vi "niFpgaMeanVarStdInsideSCTL.vi"(0 "input data":fxp<+/-,32,1>, 1 "reset":bool, 9 "input valid":bool, 12 "ready for output":bool=TRUE) -> (4 "mean":fxp<+/-,32,1> format="%.32g", 6 "standard deviation":fxp<+,32,1> format="%.32g", 8 "variance":fxp<+,63,1> format="%.63g", 10 "output valid":bool, 14 "ready for input":bool)   [LabVIEW 2017]
uses:
  <vilib>/rvi/FXPMathLib/basic elements/FxpIntAccumulator/subVIs/nifxpmath_IntAccumulator_SimConfig.ctl
  <vilib>/rvi/FXPMathLib/basic elements/FxpIntAccumulator/simVIs/DllFxpIntAccumulator_sub.vi
  <vilib>/rvi/FXPMathLib/basic elements/FxpIntAccumulator/XNode/nifxpmath_IntAccumulator.xnode
  <vilib>/fxp/LVFixedPointOverflowPolicyTypeDef.ctl
  <vilib>/rvi/FXPMathLib/FxpMul/XNode/nifxpmath_Multiplier.xnode
  <vilib>/rvi/FXPMathLib/FxpSqrt/XNode/nifxpmath_Sqrt.xnode
  <vilib>/rvi/FXPMathLib/FxpSqrt/simVIs/DllSqrtTemp_sub.vi
  <vilib>/rvi/FXPMathLib/FxpSqrt/subVIs/nifxpmath_Sqrt_SimConfig.ctl
  <vilib>/rvi/FXPMathLib/sim/FxpSim.dll
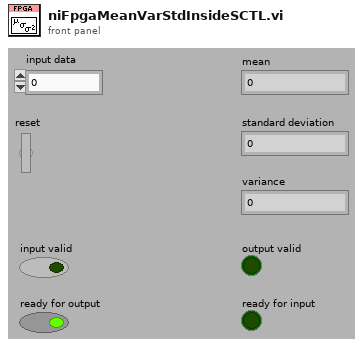
[diagram p1: front panel]
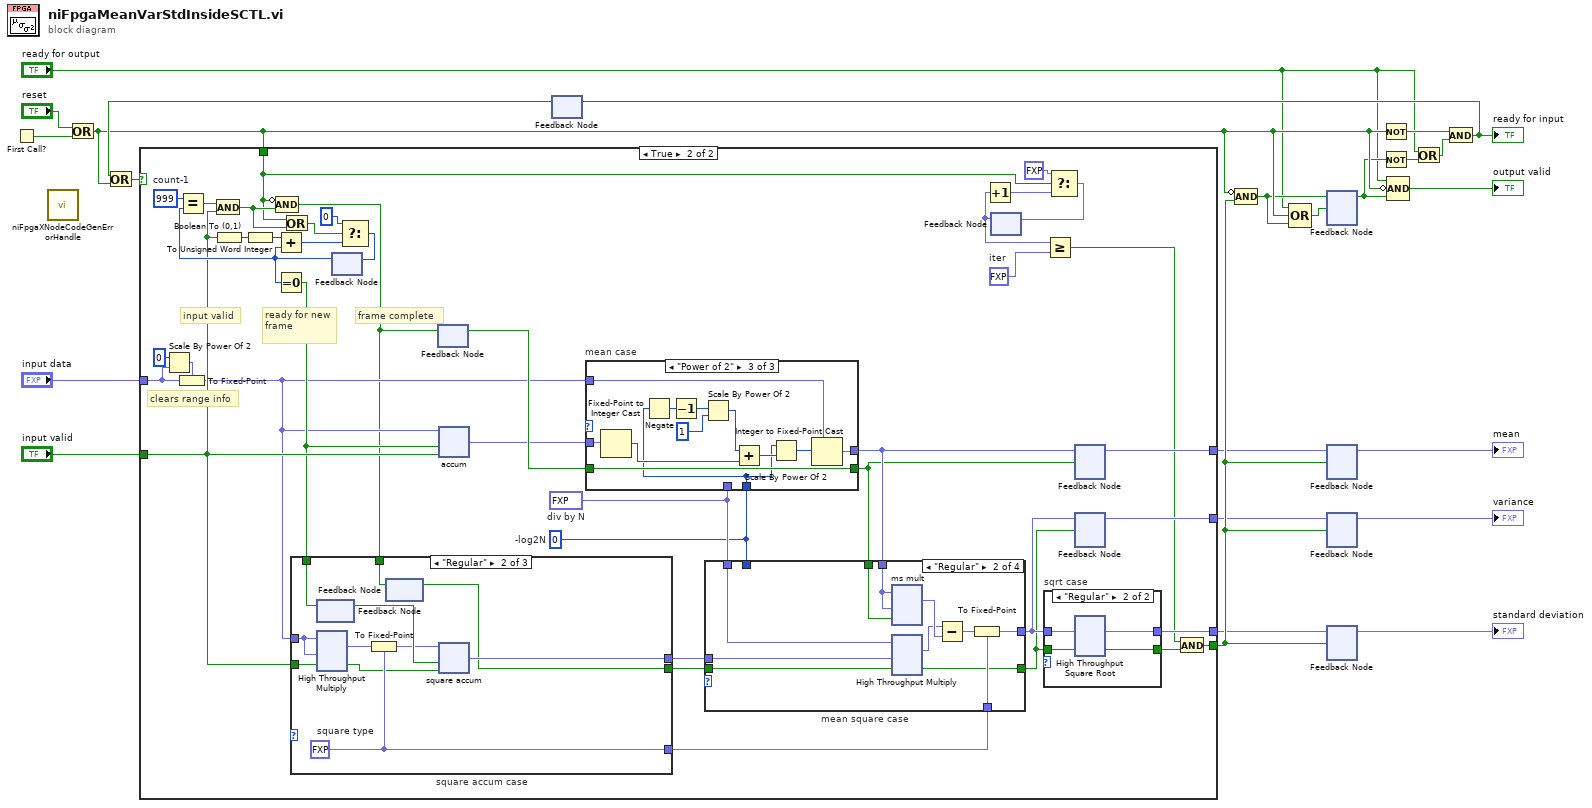
[diagram p0: block diagram]
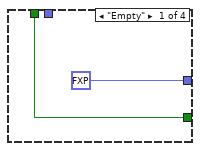
[diagram p3: hidden frame]
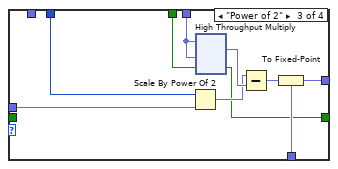
[diagram p4: hidden frame]
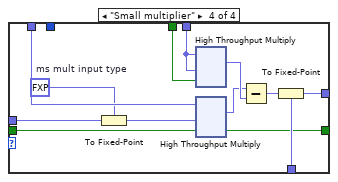
[diagram p5: hidden frame]
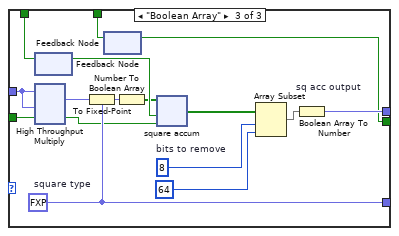
[diagram p7: hidden frame]
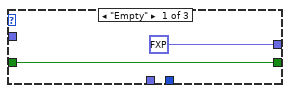
[diagram p8: hidden frame]
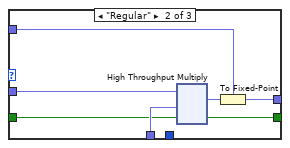
[diagram p9: hidden frame]
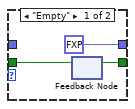
[diagram p10: hidden frame]
diagram:
  n1 = First Call?() -> (First Call?: T/F=w21:bool)
  n2 = call <vilib>:"niFpgaXNodeCodeGenErrorHandle.vi"() -> ()  [unwired: 1 in]
  n3 = Or(x="reset", y=w21) -> (x .or. y?=w7:bool)
  n4 = feedback #1() -> (w9:bool)  [unwired: 1 in]
  n5 = Or(x=w9, y=w7) -> (x .or. y?=w10:bool)
  n6 = case shown="True" w10 {
    tunnel: "input valid" -> [_ w56]
    tunnel: w7 -> [_ w49]
    tunnel: [_ w28] -> w15
    tunnel: [_ w43] -> w14
    tunnel: [_ w42] -> w13
    tunnel: [_ w36] -> w12
    tunnel: "input data" -> [_ w24]
    frame False {
    }
    frame True {
      w35 = i8 0  # -log2N
      w51 = fxp<+,6,6> 39.0  # iter
      w41 = fxp<+,18,-9> 0.0010000020265579224  # div by N
      w47 = u16 999  # count-1
      # "clears range info"
      # "frame complete"
      # "ready for new frame"
      # "input valid"
      n7 = Scale By Power Of 2(n=0, x=w24) -> (x*2^n=w25:fxp<+/-,32,1>)
      n8 = To Fixed-Point(fixed-point type=w25, number=w24) -> (fixed-point=w34:fxp<+/-,32,1>)
      n9 = Boolean To (0,1)(Boolean=w56) -> (0, 1=w63:i16)
      n10 = To Unsigned Word Integer(number=w63) -> (unsigned 16bit integer=w46:u16)
      n11 = feedback #2() -> (w59:u16)  [unwired: 1 in]
      n12 = Equal?(x=w47, y=w59) -> (x = y?=w61:bool)
      n13 = And(x=w61, y=w56) -> (x .and. y?=w57:bool)
      n14 = Compound Arithmetic op=AND(invert w49, w57) -> (w30:bool)
      n15 = Add(x=w46, y=w59) -> (x+y=w62:u16)
      n16 = Equal To 0?(x=w59) -> (x = 0?=w55:bool)
      n17 = Or(x=w49, y=w57) -> (x .or. y?=w58:bool)
      n18 = case "square accum case" shown="\"Regular\"" {
        selector: _ -> [_ _ _]
        tunnel: w56 -> [_ w137 w180]
        tunnel: w55 -> [_ w136 w179]
        tunnel: w34 -> [_ w135 w178]
        tunnel: [_ w134 w177] -> w45
        tunnel: [_ w127 w165] -> w40
        tunnel: [_ w129 w167] -> w39
        tunnel: w30 -> [_ w128 w166]
        frame "Empty" {
        }
        frame "Regular" {
          w134 = fxp<+,31,1> 0.0  # square type
          n19 = feedback-in #3(w136) -> ()
          n20 = feedback #3() -> (w132:bool)  [unwired: 1 in]
          n21 = xnode "High Throughput Multiply"("x"=w135, "y"=w135, "input valid"=w137) -> ("x*y"=w131:fxp<+/-,64,2>, "output valid"=w133:bool)  [unwired: 1 in, 1 out]
          n22 = To Fixed-Point(fixed-point type=w134, number=w131) -> (fixed-point=w130:fxp<+,31,1>)
          n23 = feedback-in #4(w128) -> ()
          n24 = feedback #4() -> (w127:bool)  [unwired: 1 in]
          n25 = xnode "square accum"("x"=w130, "load (F)"=w132, "enable (T)"=w133) -> ("s"=w129:fxp<+,41,11>)  [unwired: 2 in, 1 out]
        }
        frame "Boolean Array" {
          w171 = 8  # bits to remove
          w177 = fxp<+,63,1> 0.0  # square type
          n26 = feedback-in #5(w179) -> ()
          n27 = feedback #5() -> (w175:bool)  [unwired: 1 in]
          n28 = xnode "High Throughput Multiply"("x"=w178, "y"=w178, "input valid"=w180) -> ("x*y"=w174:fxp<+/-,64,2>, "output valid"=w176:bool)  [unwired: 1 in, 1 out]
          n29 = To Fixed-Point(fixed-point type=w177, number=w174) -> (fixed-point=w173:fxp<+,63,1>)
          n30 = feedback-in #6(w166) -> ()
          n31 = feedback #6() -> (w165:bool)  [unwired: 1 in]
          n32 = Number To Boolean Array(number=w173) -> (Boolean array=w172:bool[])
          n33 = xnode "square accum"("x"=w172, "load (F)"=w175, "enable (T)"=w176) -> ("s"=w168:bool[])  [unwired: 2 in, 1 out]
          n34 = Array Subset(array=w168, index=w171, length=64) -> (w169:bool[])
          n35 = Boolean Array To Number "sq acc output"(Boolean array=w169) -> (number=w167:fxp<+,64,10>)
        }
      }
      n36 = Select(t=u16 0, s=w58, f=w62) -> (s? t:f=w48:u16)
      n37 = feedback-in #2(w48) -> ()
      n38 = feedback-in #7(w30) -> ()
      n39 = feedback #7() -> (w38:bool)  [unwired: 1 in]
      n40 = xnode "accum"("x"=w34, "load (F)"=w55, "enable (T)"=w56) -> ("s"=w37:fxp<+/-,42,11>)  [unwired: 2 in, 1 out]
      n41 = case "mean case" shown="\"Power of 2\"" {
        selector: _ -> [_ _ _]
        tunnel: w34 -> [_ w211 w213]
        tunnel: w41 -> [_ w210 _]
        tunnel: w38 -> [w204 w209 w223]
        tunnel: w37 -> [_ w208 w215]
        tunnel: [w204 w207 w223] -> w31
        tunnel: [fxp<+/-,16,1> 0.0 ("input data") w206 w214] -> w32
        tunnel: w35 -> [_ _ w212]
        frame "Empty" {
        }
        frame "Regular" {
          n42 = xnode "High Throughput Multiply"("x"=w208, "y"=w210, "input valid"=w209) -> ("x*y"=w205:fxp<+/-,60,2>, "output valid"=w207:bool)  [unwired: 1 in, 1 out]
          n43 = To Fixed-Point(fixed-point type=w211, number=w205) -> (fixed-point=w206:fxp<+/-,32,1>)
        }
        frame "Power of 2" {
          n44 = Fixed-Point to Integer Cast(1:w215) -> (0:w218:i64)
          n45 = Negate(x=w212) -> (-x=w222:i8)
          n46 = Decrement(x=w222) -> (x-1=w221:i8)
          n47 = Scale By Power Of 2(n=w221, x=i64 1 ("x-1")) -> (x*2^n=w219:i64)
          n48 = Add(x=w219, y=w218) -> (x+y=w216:i64)
          n49 = Scale By Power Of 2(n=w212, x=w216) -> (x*2^n=w217:i64)
          n50 = Integer to Fixed-Point Cast(fixed-point type=w213, integer=w217) -> (fixed-point=w214:fxp<+/-,32,1>)
        }
      }
      n51 = case "mean square case" shown="\"Regular\"" {
        selector: _ -> [_ _ _ _]
        tunnel: w45 -> [_ w103 w113 w126]
        tunnel: [w91 w102 w104 w125] -> w33
        tunnel: [fxp<+,31,1> 0.0 ("square type") w101 w112 w124] -> w44
        tunnel: w41 -> [_ w100 _ w123]
        tunnel: w40 -> [_ w99 _ w122]
        tunnel: w39 -> [_ w98 w111 w121]
        tunnel: w35 -> [_ _ w110 _]
        tunnel: w32 -> [_ w93 w108 w118]
        tunnel: w31 -> [w91 w94 w109 w117]
        frame "Empty" {
        }
        frame "Regular" {
          n52 = xnode ("ms mult")("x"=w93, "y"=w93, "input valid"=w94) -> ("x*y"=w97:fxp<+/-,64,2>)  [unwired: 1 in, 2 out]
          n53 = xnode ("High Throughput Multiply")("x"=w100, "y"=w98, "input valid"=w99) -> ("x*y"=w96:fxp<+,64,2>, "output valid"=w102:bool)  [unwired: 1 in, 1 out]
          n54 = Subtract(x=w96, y=w97) -> (x-y=w95:fxp<+/-,64,4>)
          n55 = To Fixed-Point(fixed-point type=w103, number=w95) -> (fixed-point=w101:fxp<+,63,1>)
        }
        frame "Power of 2" {
          n56 = Scale By Power Of 2(n=w110, x=w111) -> (x*2^n=w106:fxp<+,64,11>)
          n57 = xnode "High Throughput Multiply"("x"=w108, "y"=w108, "input valid"=w109) -> ("x*y"=w107:fxp<+/-,64,2>, "output valid"=w104:bool)  [unwired: 1 in, 1 out]
          n58 = Subtract(x=w106, y=w107) -> (x-y=w105:fxp<+/-,64,13>)
          n59 = To Fixed-Point(fixed-point type=w113, number=w105) -> (fixed-point=w112:fxp<+,63,1>)
        }
        frame "Small multiplier" {
          w119 = fxp<+,34,10> 0.0  # ms mult input type
          n60 = To Fixed-Point(fixed-point type=w119, number=w121) -> (fixed-point=w120:fxp<+,34,10>)
          n61 = xnode ("High Throughput Multiply")("x"=w118, "y"=w118, "input valid"=w117) -> ("x*y"=w116:fxp<+/-,64,2>)  [unwired: 1 in, 2 out]
          n62 = xnode ("High Throughput Multiply")("x"=w123, "y"=w120, "input valid"=w122) -> ("x*y"=w115:fxp<+,52,1>, "output valid"=w125:bool)  [unwired: 1 in, 1 out]
          n63 = Subtract(x=w115, y=w116) -> (x-y=w114:fxp<+/-,64,3>)
          n64 = To Fixed-Point(fixed-point type=w126, number=w114) -> (fixed-point=w124:fxp<+,63,1>)
        }
      }
      n65 = feedback #8() -> (w50:fxp<+,6,6>)  [unwired: 1 in]
      n66 = Increment(x=w50) -> (x+1=w53:fxp<+,6,6>)
      n67 = case "sqrt case" shown="\"Regular\"" {
        selector: _ -> [_ _]
        tunnel: [w224 w230] -> w29
        tunnel: w33 -> [w225 w229]
        tunnel: w44 -> [_ w228]
        tunnel: [fxp<+,16,1> 0.0 ("sqrt(x)") w227] -> w42
        frame "Empty" {
          n68 = feedback-in #9(w225) -> ()
          n69 = feedback #9() -> (w224:bool)  [unwired: 1 in]
        }
        frame "Regular" {
          n70 = xnode ("High Throughput Square Root")("x"=w228, "input valid"=w229) -> ("sqrt(x)"=w227:fxp<+,32,1>, "output valid"=w230:bool)  [unwired: 1 in, 1 out]
        }
      }
      n71 = Greater Or Equal?(x=w50, y=w51) -> (x >= y?=w27:bool)
      n72 = Select(t=fxp<+,1,1> 0.0, s=w49, f=w53) -> (s? t:f=w52:fxp<+,6,6>)
      n73 = feedback-in #8(w52) -> ()
      n74 = feedback-in #10(w32, w31) -> ()
      n75 = feedback #10() -> (w36:fxp<+/-,32,1>)  [unwired: 1 in]
      n76 = feedback-in #11(w44, w33) -> ()
      n77 = feedback #11() -> (w43:fxp<+,63,1>)  [unwired: 1 in]
      n78 = And(x=w27, y=w29) -> (x .and. y?=w28:bool)
    }
  }
  n79 = Compound Arithmetic op=AND(invert w7, w15) -> (w6:bool)
  n80 = Compound Arithmetic op=OR("ready for output", w7, w6) -> (w5:bool)
  n81 = feedback-in #12(w6, w5) -> ()
  n82 = feedback #12() -> (w4:bool)  [unwired: 1 in]
  n83 = feedback-in #13(w12, w15) -> ()
  n84 = feedback #13() -> (→"mean":fxp<+/-,32,1>)  [unwired: 1 in]
  n85 = feedback-in #14(w14, w15) -> ()
  n86 = feedback #14() -> (→"variance":fxp<+,63,1>)  [unwired: 1 in]
  n87 = feedback-in #15(w13, w15) -> ()
  n88 = feedback #15() -> (→"standard deviation":fxp<+,32,1>)  [unwired: 1 in]
  n89 = Not(x=w7) -> (.not. x?=w18:bool)
  n90 = Not(x=w4) -> (.not. x?=w2:bool)
  n91 = Compound Arithmetic op=AND("ready for output", invert w7, w4) -> (→"output valid":bool)
  n92 = Or(x="ready for output", y=w2) -> (x .or. y?=w1:bool)
  n93 = And(x=w18, y=w1) -> (x .and. y?=w8:bool)
  "ready for input" <- w8
  n94 = feedback-in #1(w8) -> ()
